vi "fgv_latlong-sim.vi"(7 "cmd":T1, 10 "latlong-c":cluster{"lat":dbl, "long":dbl}, 11 "latlong a":dbl[](array[numeric])) -> (2 "latlong-c out":cluster{"lat":dbl, "long":dbl}, 3 "latlong out":dbl[](array[numeric]))   [LabVIEW 2019]
uses:
  Ctrl/cmd_common.ctl
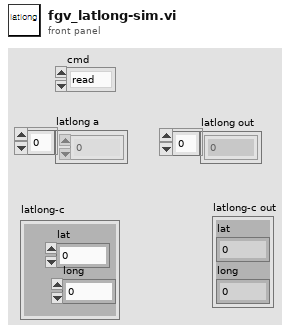
[diagram p1: front panel]
types:
  T1 = typedef "cmd_common.ctl" = enum16{"read", "write"}
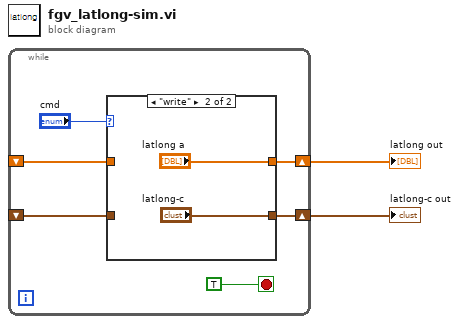
[diagram p0: block diagram]
diagram:
  n1 = while {
    shift-right: [w6] -> w2
    shift-left: _ -> [w5]
    shift-right: [w4] -> w1
    shift-left: _ -> [w3]
    stop <- TRUE stop-if-true
    n2 = case shown="\"write\"" "cmd" {
      tunnel: [w10 "latlong a"] -> w6
      tunnel: w5 -> [w10 _]
      tunnel: [w9 "latlong-c"] -> w4
      tunnel: w3 -> [w9 _]
      frame "read", Default {
      }
      frame "write" {
      }
    }
  }
  "latlong out" <- w2
  "latlong-c out" <- w1
